vi "Flatten.vi"(8 "error in":errorcluster, 9 "Data":T1) -> (0 "error out":errorcluster, 2 "Buffer":u8[](array[numeric]) format="%.0x")   [LabVIEW 2020, in "StringData.lvlib"]
uses:
  StringData.lvlib
  Data.ctl
  lv-protoc/LV-Proto/LV-Proto.lvlib
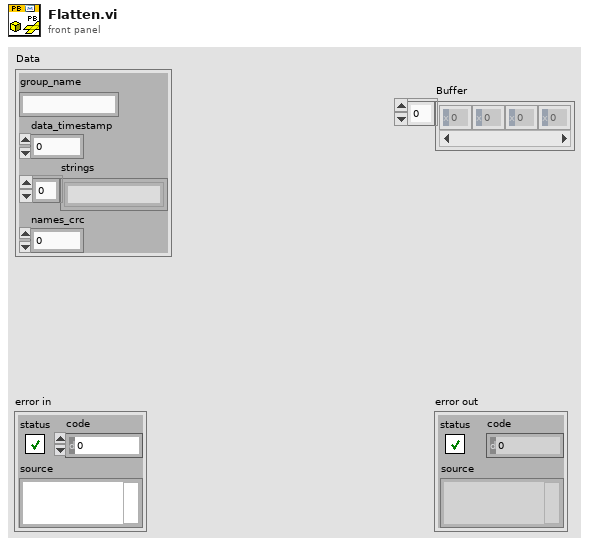
[diagram p1: front panel]
types:
  T1 = typedef "StringData.lvlib/Data.ctl" = cluster{"group_name":string, "data_timestamp":i64, "strings":string[], "names_crc":u32}
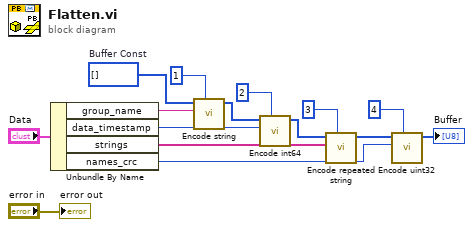
[diagram p0: block diagram]
diagram:
  w13 = u8[] []  # Buffer Const
  n1 = Unbundle By Name("Data") -> ("group_name"=w11:string, "data_timestamp"=w8:i64, "strings"=w5:string[], "names_crc"=w2:u32)
  n2 = call "Encode string.vi"("Field Number"=1, "string"=w11, "Buffer in"=w13) -> ("Buffer"=w10:u8[])  [unwired: 8 in]
  n3 = call "Encode int64.vi"("Field Number"=2, "int64"=w8, "Buffer in"=w10) -> ("Buffer"=w7:u8[])  [unwired: 8 in]
  n4 = call "Encode repeated string.vi"("Field Number"=3, "string"=w5, "Buffer in"=w7) -> ("Buffer"=w4:u8[])  [unwired: 8 in]
  n5 = call "Encode uint32.vi"("Field Number"=4, "uint32"=w2, "Buffer in"=w4) -> ("Buffer"=→"Buffer":u8[])  [unwired: 8 in]
  "error out" <- "error in"
